vi "objectCreationSequence.vi"(7 "Shared Resource (F)":bool, 8 "error in (no error)":errorcluster, 10 "Subsystem Name (optional)":string, 11 "SMO in":refnum<class "SMO.lvclass">) -> (0 "error out":errorcluster, 3 "SMO out":refnum<class "SMO.lvclass">)   [LabVIEW 2021, in "smo.lvlib" / "SMO.lvclass"]
uses:
  SMO.lvclass
  SMO.lvclass/SMO.ctl
  Support/Attribute/Attribute.lvclass/Attribute.ctl
  Support/Attribute/Read AttrName.vi
  ReftoDVR--SMO.vi
  GetVariant(Attr).vi
  Support/Attribute.Dependencies/Attribute.Dependencies.lvclass
  C:/Repositories/SMO/src/Support/Attribute/Attribute.lvclass
  Support/Attribute.Identity/Attribute.Identity.lvclass
  <vilib>/Utility/LVClass/Get LV Class Name.vi
  <vilib>/Utility/error.llb/Error Cluster From Error Code.vi
  SetVariant(Attr).vi
  Support/Attribute/Attribute.lvclass
  Registry/Registry-SMO.lvclass
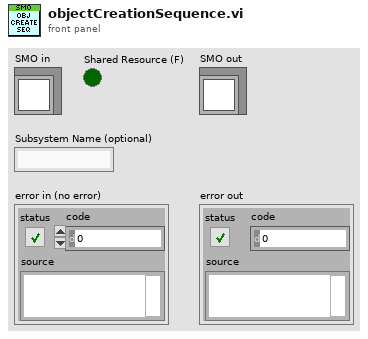
[diagram p1: front panel]
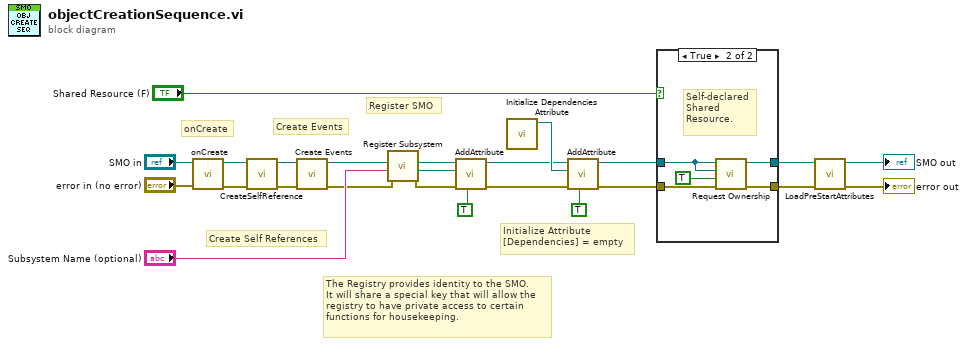
[diagram p0: block diagram]
diagram:
  # "Initialize Attribute\n[Dependencies] = empty"
  # "The Registry provides identity to the SMO.\nIt will share a special key that will allow the\nregistry to have private access to certain\nfunctions for housekeeping."
  # "Create Self References"
  # "Register SMO"
  # "Create Events"
  # "onCreate"
  n1 = call-dynamic "onCreate.vi"("error in (no error)"="error in (no error)", "SMO"="SMO in") -> ("error out"=w17:errorcluster, "SMO out"=w15:refnum<class "SMO.lvclass">)  [unwired: 8 in]
  n2 = call-dynamic "CreateSelfReference.vi"("error in (no error)"=w17, "SMO"=w15) -> ("error out"=w18:errorcluster, "SMO out"=w16:refnum<class "SMO.lvclass">)  [unwired: 8 in]
  n3 = call "Create Events.vi"("error in (no error)"=w18, "SMO"=w16) -> ("error out"=w9:errorcluster, "SMO out"=w8:refnum<class "SMO.lvclass">)  [unwired: 8 in]
  n4 = call "Register Subsystem.vi"("error in (no error)"=w9, "Subsystem Name (optional)"="Subsystem Name (optional)", "Unregistered SMO"=w8) -> ("error out"=w14:errorcluster, "Attribute.Identity"=w19:refnum<class "Attribute.Identity.lvclass">, "Registered SMO"=w13:refnum<class "SMO.lvclass">)  [unwired: 6 in]
  n5 = call "AddAttribute.vi"("Overwrite? (F)"=TRUE, "error in (no error)"=w14, "Attribute"=w19, "SMO in"=w13) -> ("error out"=w23:errorcluster, "SMO out"=w20:refnum<class "SMO.lvclass">)  [unwired: 6 in]
  n6 = call "Initialize Dependencies Attribute.vi"() -> ("Attribute.Dependencies"=w21:refnum<class "Attribute.Dependencies.lvclass">)  [unwired: 11 in]
  n7 = call "AddAttribute.vi"("Overwrite? (F)"=TRUE, "error in (no error)"=w23, "Attribute"=w21, "SMO in"=w20) -> ("error out"=w6:errorcluster, "SMO out"=w5:refnum<class "SMO.lvclass">)  [unwired: 6 in]
  n8 = case shown="True" "Shared Resource (F)" {
    tunnel: [w26 w31] -> w1
    tunnel: w6 -> [w25 w30]
    tunnel: [w25 w29] -> w3
    tunnel: w5 -> [w26 w28]
    frame False {
    }
    frame True {
      # "Self-declared\nShared\nResource."
      n9 = call "Request Ownership.vi"("error in (no error)"=w30, "Shared Resource"=TRUE, "Dependency"=w28, "SMO in"=w28) -> ("error out"=w29:errorcluster, "SMO out"=w31:refnum<class "SMO.lvclass">)  [unwired: 5 in, 1 out]
    }
  }
  n10 = call "LoadPreStartAttributes.vi"("error in (no error)"=w3, "SMO in"=w1) -> ("error out"=→"error out":errorcluster, "SMO out"=→"SMO out":refnum<class "SMO.lvclass">)  [unwired: 8 in]
